vi "Send Unregister.vi"(8 "Error In":errorcluster, 10 "Registrant Address":refnum<class "Message Enqueuer.lvclass">, 11 "Event Source Address":refnum<class "Message Enqueuer.lvclass">) -> (0 "Error Out":errorcluster, 3 "Event Source Address Out":refnum<class "Message Enqueuer.lvclass">)   [LabVIEW 2016, in "Event Source.lvlib" / "Unregister Msg.lvclass"]
doc: "Send an unregister message to the Event Source Actor. \n\n<b>IMPORTANT</b> - All registrants should have this method in their <b>Stop Core.vi</b>"
uses:
  Unregister Msg.lvclass
  <vilib>/ActorFramework/Message Enqueuer/Message Enqueuer.lvclass
  C:/Program Files (x86)/National Instruments/LabVIEW 2016/vi.lib/ActorFramework/Message/Message.lvclass
  Unregister Msg.lvclass/Unregister Msg.ctl
  <vilib>/ActorFramework/Message Enqueuer/Message Enqueuer.lvclass/Message Enqueuer.ctl
  <vilib>/ActorFramework/Message Priority Queue/Priority Enqueue.vi
  <resource>/AFDebug/Generate Trace for Message.vi
  <vilib>/Utility/LVClass/Get LV Class Name.vi
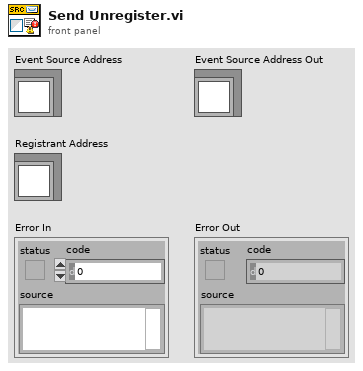
[diagram p1: front panel]
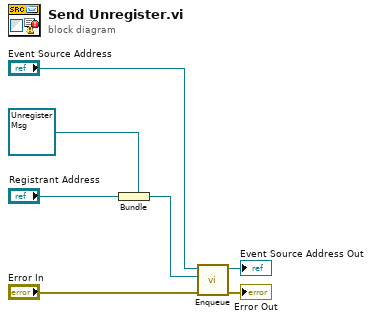
[diagram p0: block diagram]
diagram:
  n1 = Bundle(cluster=refnum<class "Unregister Msg.lvclass"> refnum ("Message Type"), "Registrant Address") -> (w3:refnum<class "Unregister Msg.lvclass">)
  n2 = call <vilib>:"Enqueue.vi"("error in (no error)"="Error In", "Message"=w3, "Message Enqueuer in"="Event Source Address") -> ("error out"=→"Error Out":errorcluster, "Message Enqueuer out"=→"Event Source Address Out":refnum<class "Message Enqueuer.lvclass">)  [unwired: 7 in]
